vi "Check Power Data.vi"(4 "PS Channel Control":i32, 6 "station name":string, 7 "power supply type":T1, 8 "Error Table In":string[][](table), 9 "station idx":i32=4, 10 "Power Supply Voltage":dbl, 11 "Power Supply Comm Port":refnum<visa-resource-name>="COM1") -> (0 "Error Table Out":string[][](array[string]), 2 "Actual Voltage":dbl, 3 "Pass?":bool)   [LabVIEW 2018]
uses:
  05.UserVI's/Lambda Power/power supply types.ctl
  ZUP_Current/Def Ctrl/CMD Type.ctl
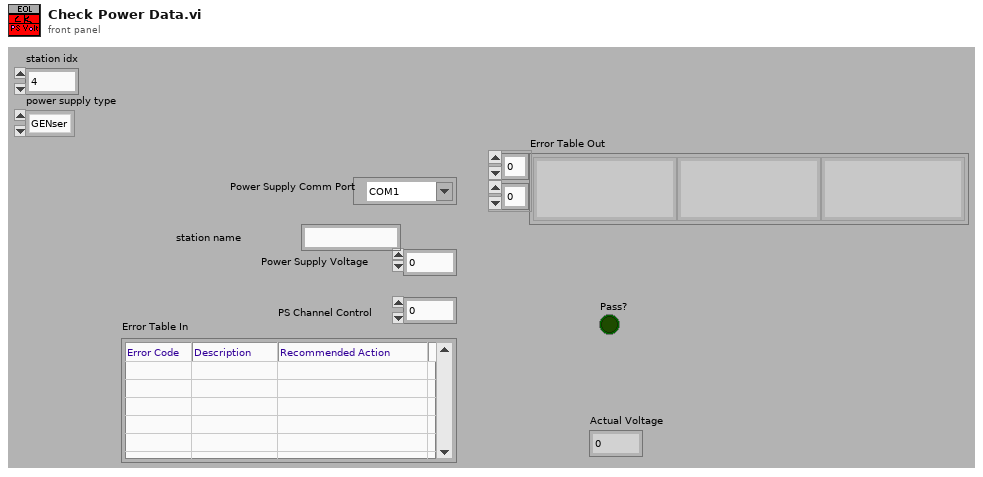
[diagram p1: front panel]
types:
  T1 = typedef "power supply types.ctl" = enum16{"GENser", "ZUPser", "GENeth", "Manual", "ITECH"}
  T2 = cluster{"Set？":bool, "Power Supply Voltage":dbl, "station name":string, "Max Voltage":dbl, "Min Voltage":dbl, "PS Channel Control":i32, "Power Supply Comm Port":refnum<visa-resource-name>, "Error String":string, "Actual Voltage":dbl, "Start Timer":u32, "Pass?":bool, "station idx":i32, "power supply type":T1}
  T3 = typedef "CMD Type.ctl" = enum16{"Default", "SetADR", "SetRMT", "SetVOL", "SetCUR", "SetOUT", "CheckREV", "CheckRMT", "CheckVOL", "CkeckCUR", "CheckOUT"}
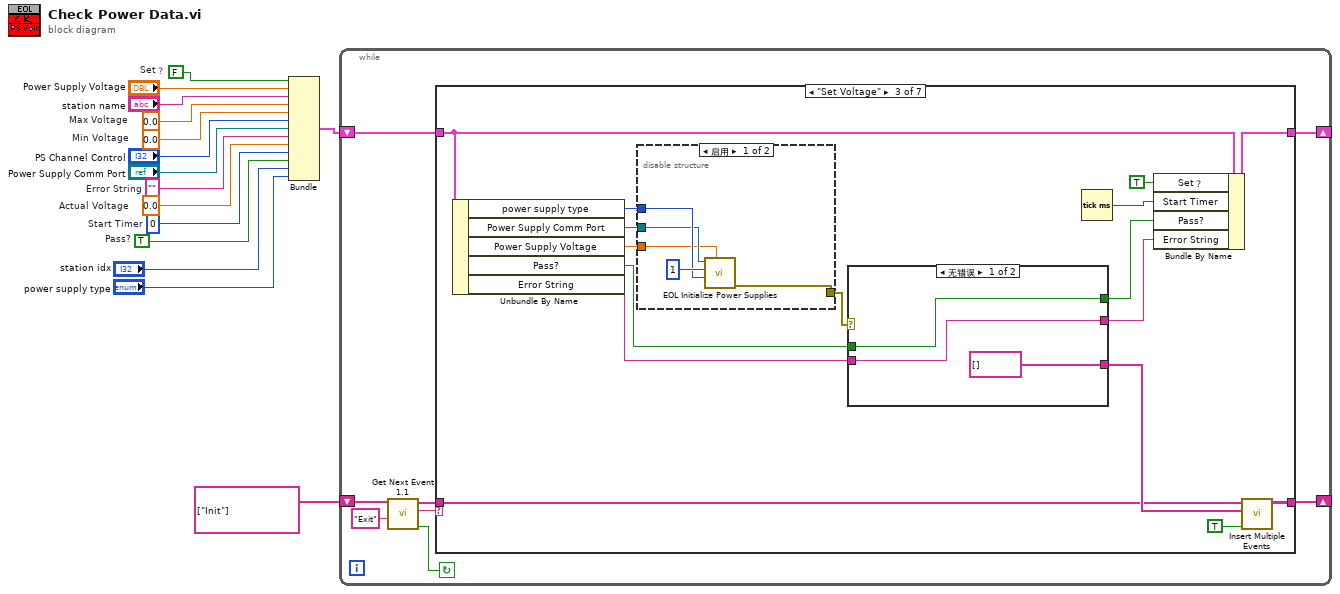
[diagram p0: block diagram]
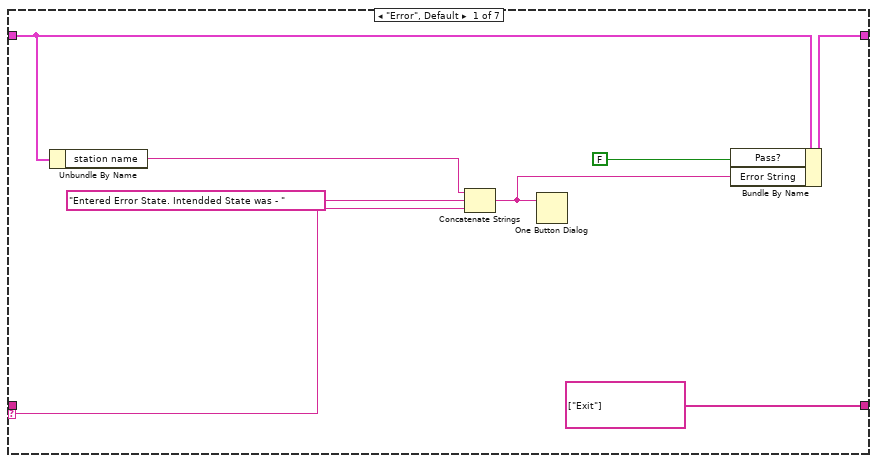
[diagram p2: hidden frame]
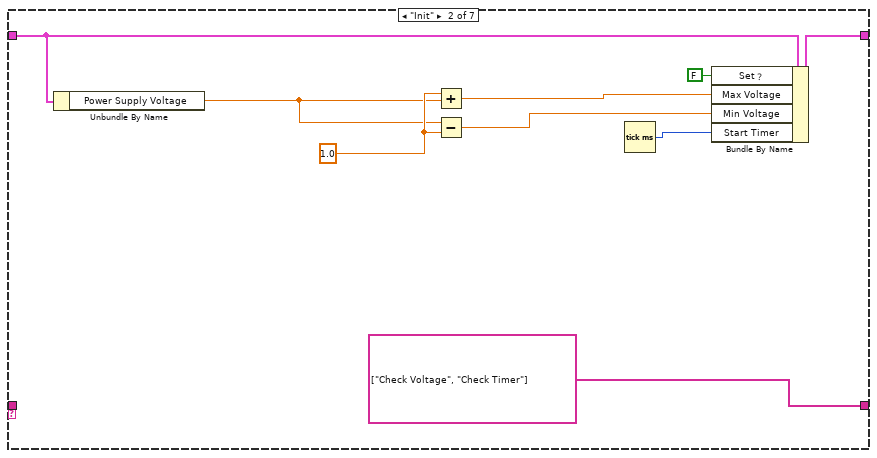
[diagram p3: hidden frame]
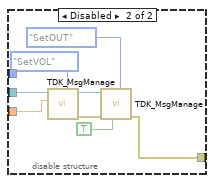
[diagram p4: hidden frame]
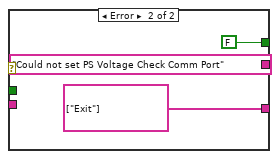
[diagram p5: hidden frame]
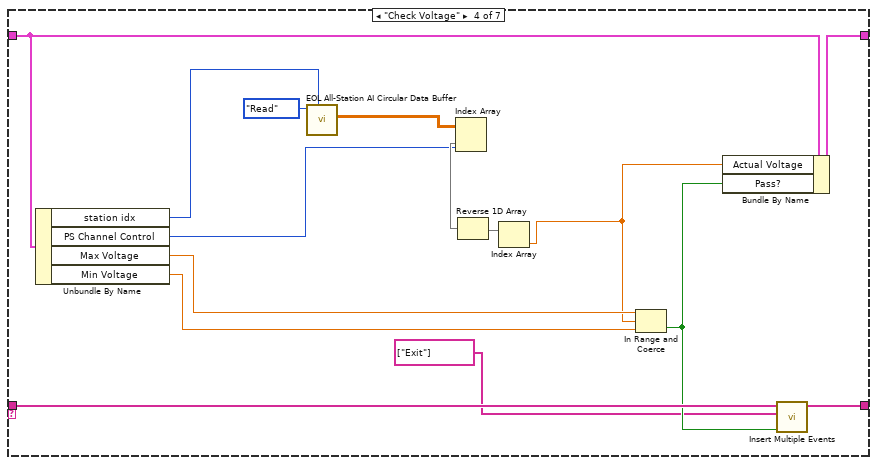
[diagram p6: hidden frame]
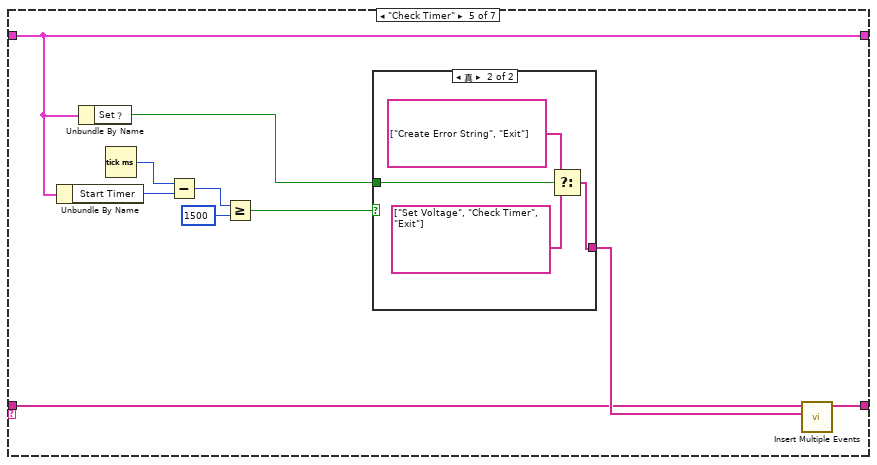
[diagram p7: hidden frame]
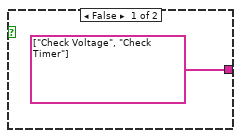
[diagram p8: hidden frame]
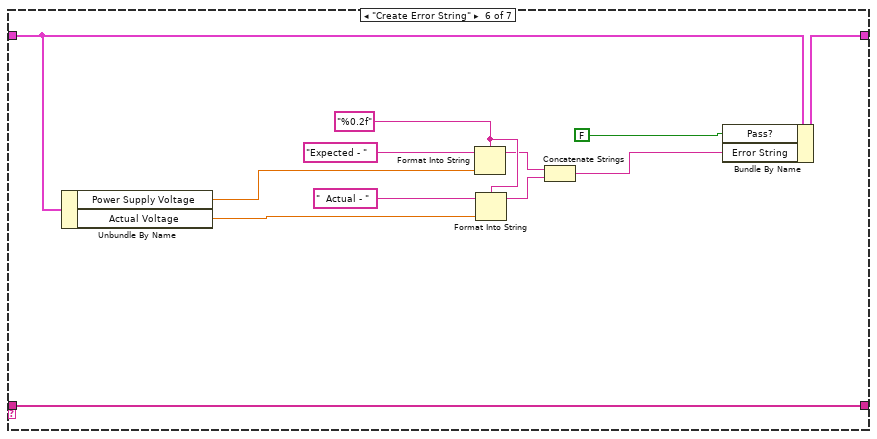
[diagram p9: hidden frame]
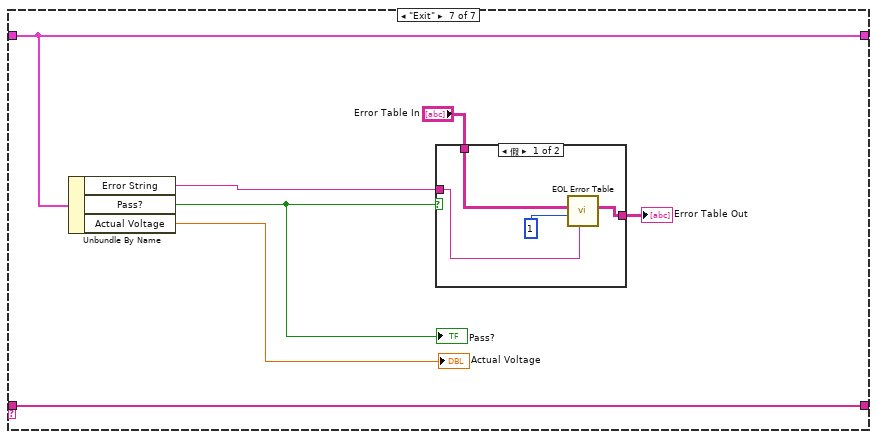
[diagram p10: hidden frame]
diagram:
  w1 = FALSE  # Set？
  w4 = TRUE  # Pass?
  w5 = u32 0  # Start Timer
  w6 = 0.0  # Actual Voltage
  w7 = ""  # Error String
  w11 = 0.0  # Max Voltage
  w10 = 0.0  # Min Voltage
  n1 = Bundle("Set？"=w1, "Power Supply Voltage"="Power Supply Voltage", "station name"="station name", "Max Voltage"=w11, "Min Voltage"=w10, "PS Channel Control"="PS Channel Control", "Power Supply Comm Port"="Power Supply Comm Port", "Error String"=w7, "Actual Voltage"=w6, "Start Timer"=w5, "Pass?"=w4, "station idx"="station idx", "power supply type"="power supply type") -> (w12:T2)  [unwired: 1 in]
  n2 = while {
    shift-right: [w19] -> _
    shift-left: string[] ["Init"] ("event queue out") -> [w18]
    shift-right: [w16] -> _
    shift-left: w12 -> [w17]
    stop <- w23 continue-if-true
    n3 = call "Get Next Event 1.1.vi"("Exit Event"="Exit", "event queue in"=w18) -> ("Condition (Exit:F)"=w23:bool, "next event"=w21:string, "event queue out"=w20:string[])  [unwired: 6 in, 1 out]
    n4 = case shown="\"Set Voltage\"" w21 {
      selector: w21 -> [w30 _ _ _ _ _ _]
      tunnel: w20 -> [_ _ w54 w84 w93 w117 w124]
      tunnel: [string[] ["Exit"] ("event queue out") string[] ["Check Voltage", "Check Timer"] ("event queue out") w56 w85 w94 w117 w124] -> w19
      tunnel: w17 -> [w28 w37 w52 w87 w92 w116 w121]
      tunnel: [w27 w36 w51 w86 w92 w115 w121] -> w16
      frame "Error", Default {
        n5 = Unbundle By Name(w28) -> ("station name"=w24:string)
        n6 = Concatenate Strings(w24, "Entered Error State. Intendded State was - " ("string"), w30) -> (w25:string)
        n7 = One Button Dialog(message=w25) -> ()  [unwired: 1 in, 1 out]
        n8 = Bundle By Name(cluster=w28, "Pass?"=FALSE, "Error String"=w25) -> (w27:T2)
      }
      frame "Init" {
        w39 = 1.0 ("x")
        n9 = Unbundle By Name(w37) -> ("Power Supply Voltage"=w38:dbl)
        n10 = Add(x=w39, y=w38) -> (x+y=w35:dbl)
        n11 = Subtract(x=w38, y=w39) -> (x-y=w34:dbl)
        n12 = Tick Count (ms)() -> (millisecond timer value=w33:u32)
        n13 = Bundle By Name(cluster=w37, "Set？"=FALSE, "Max Voltage"=w35, "Min Voltage"=w34, "Start Timer"=w33) -> (w36:T2)
      }
      frame "Set Voltage" {
        n14 = Unbundle By Name(w52) -> ("power supply type"=w45:T1, "Power Supply Comm Port"=w44:refnum<visa-resource-name>, "Power Supply Voltage"=w43:dbl, "Pass?"=w47:bool, "Error String"=w49:string)
        n15 = disable-structure shown="启用" {
          disable-tunnel: w45 -> [w60 _]
          disable-tunnel: w44 -> [w59 w68]
          disable-tunnel: w43 -> [w58 w69]
          disable-tunnel: [w57 w62] -> w42
          frame Enabled {
            n16 = call "EOL Initialize Power Supplies.vi"("Volt Limit"=w58, "power supply model"=w60, "No. of Power Supplies"=1, "VISA resource name"=w59) -> ("error out"=w57:errorcluster)  [unwired: 7 in]
          }
          frame Disabled {
            n17 = call "TDK_MsgManage.vi"("CMD Type"=CMD_Type."SetVOL", "Voltage"=w69, "VISA resource name"=w68) -> ("error out"=w66:errorcluster, "VISA resource name"=w65:refnum<visa-resource-name>)  [unwired: 5 in, 2 out]
            n18 = call "TDK_MsgManage.vi"("CMD Type"=CMD_Type."SetOUT", "OUT?"=TRUE, "error in (no error)"=w66, "VISA resource name"=w65) -> ("error out"=w62:errorcluster)  [unwired: 4 in, 3 out]
          }
        }
        n19 = case shown="无错误" w42 {
          tunnel: [string[] [] ("event queue out") string[] ["Exit"] ("event queue out")] -> w55
          tunnel: [w71 "Could not set PS Voltage Check Comm Port"] -> w50
          tunnel: w49 -> [w71 _]
          tunnel: w47 -> [w70 _]
          tunnel: [w70 FALSE ("Pass?")] -> w46
          frame No Error {
          }
          frame Error {
          }
        }
        n20 = Tick Count (ms)() -> (millisecond timer value=w48:u32)
        n21 = Bundle By Name(cluster=w52, "Set？"=TRUE, "Start Timer"=w48, "Pass?"=w46, "Error String"=w50) -> (w51:T2)
        n22 = call "Insert Multiple Events.vi"("Insert all? (T)"=TRUE, "Events to Insert"=w55, "Event queue in"=w54) -> ("Event queue out"=w56:string[])  [unwired: 4 in]
      }
      frame "Check Voltage" {
        n23 = Unbundle By Name(w87) -> ("station idx"=w79:i32, "PS Channel Control"=w78:i32, "Max Voltage"=w89:dbl, "Min Voltage"=w88:dbl)
        n24 = call "EOL All-Station AI Circular Data Buffer.vi"("station idx"=w79, "Mode"=enum16{"Initialize", "Read", "Write"}."Read") -> ("Data Read (Samp-Ro, Ch-Col)"=w81:sgl[][])  [unwired: 9 in]
        n25 = Index Array(array=w81, index (col)=w78) -> (element=w80:sgl[])  [unwired: 1 in]
        n26 = Reverse 1D Array(array=w80) -> (reversed array=w90:sgl[])
        n27 = Index Array(array=w90) -> (element=w77:sgl)  [unwired: 1 in]
        n28 = In Range and Coerce(upper limit=w89, x=w77, lower limit=w88) -> (In Range?=w83:bool)  [unwired: 1 out]
        n29 = Bundle By Name(cluster=w87, "Actual Voltage"=w77, "Pass?"=w83) -> (w86:T2)
        n30 = call "Insert Multiple Events.vi"("Insert all? (T)"=w83, "Events to Insert"=string[] ["Exit"] ("event queue out"), "Event queue in"=w84) -> ("Event queue out"=w85:string[])  [unwired: 4 in]
      }
      frame "Check Timer" {
        n31 = Unbundle By Name(w92) -> ("Start Timer"=w99:u32)
        n32 = Unbundle By Name(w92) -> ("Set？"=w91:bool)
        n33 = Tick Count (ms)() -> (millisecond timer value=w100:u32)
        n34 = Subtract(x=w100, y=w99) -> (x-y=w98:u32)
        n35 = Greater Or Equal?(x=w98, y=u32 1500) -> (x >= y?=w96:bool)
        n36 = case shown="真" w96 {
          tunnel: [string[] ["Check Voltage", "Check Timer"] ("event queue out") w102] -> w95
          tunnel: w91 -> [_ w105]
          frame False {
          }
          frame True {
            n37 = Select(t=string[] ["Create Error String", "Exit"] ("event queue out"), s=w105, f=string[] ["Set Voltage", "Check Timer", "Exit"] ("event queue out")) -> (s? t:f=w102:string[])
          }
        }
        n38 = call "Insert Multiple Events.vi"("Events to Insert"=w95, "Event queue in"=w93) -> ("Event queue out"=w94:string[])  [unwired: 5 in]
      }
      frame "Create Error String" {
        w113 = "%0.2f" ("format string")
        n39 = Unbundle By Name(w116) -> ("Power Supply Voltage"=w108:dbl, "Actual Voltage"=w107:dbl)
        n40 = Format Into String(format string=w113, initial string="Expected - ", w108) -> (resulting string=w111:string)  [unwired: 1 in, 1 out]
        n41 = Format Into String(format string=w113, initial string="  Actual - ", w107) -> (resulting string=w112:string)  [unwired: 1 in, 1 out]
        n42 = Concatenate Strings(w111, w112) -> (w106:string)
        n43 = Bundle By Name(cluster=w116, "Pass?"=FALSE, "Error String"=w106) -> (w115:T2)
      }
      frame "Exit" {
        n44 = Unbundle By Name(w121) -> ("Error String"=w119:string, "Pass?"=w120:bool, "Actual Voltage"=→"Actual Voltage":dbl)
        "Pass?" <- w120
        n45 = case shown="假" w120 {
          tunnel: "Error Table In" -> [w128 w129]
          tunnel: [w125 w129] -> w123
          tunnel: w119 -> [w127 _]
          frame False {
            n46 = call "EOL Error Table.vi"("Error Description"=w127, "Error No."=u16 1, "Error Table In"=w128) -> ("Error Table Out"=w125:string[][])  [unwired: 7 in, 1 out]
          }
          frame True {
          }
        }
        "Error Table Out" <- w123
      }
    }
  }
